vi "Demo_Single-Channel device.vi"() -> ()   [LabVIEW 2011]
doc: "This example shows how to configure a range and check that the acquired measurements are within that range using the VIs of the driver."
uses:
  <instrlib>/Thorlabs_MDT69xB/Thorlabs_MDT69xB.lvlib
panel:
  in  "Set x max Voltage(V)":dbl
  out "Get x min voltage(V)":dbl
  in  "Set x min Voltage(V)":dbl
  out "Get x max voltage(V)":dbl
  out "v limit(V)":dbl
  out "Get X voltage(V)":dbl
  in  "Set X voltage(V)":dbl
  out "?":string
  # "Device Info"
  # "Set Params"
  # "Get Params"
  # "(c) 2019 <Thorlabs>.  ALL RIGHTS RESERVED."
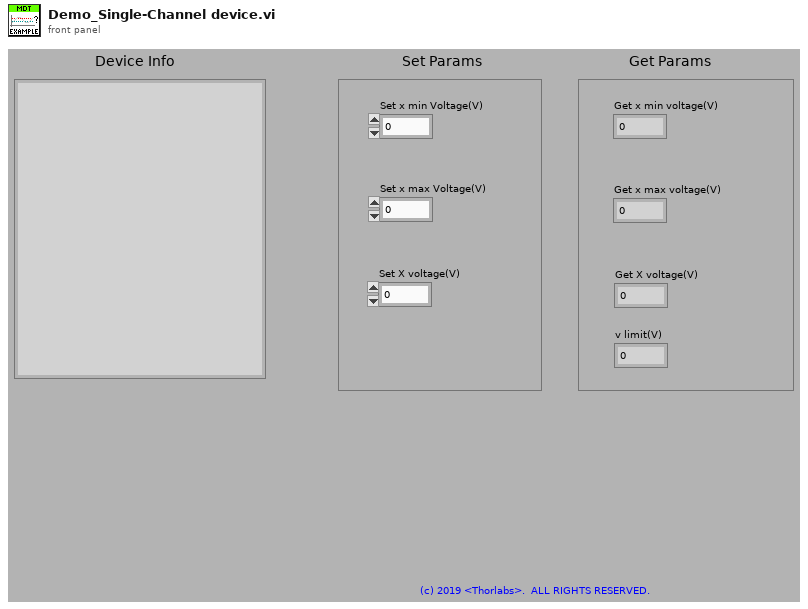
[diagram p1: front panel]
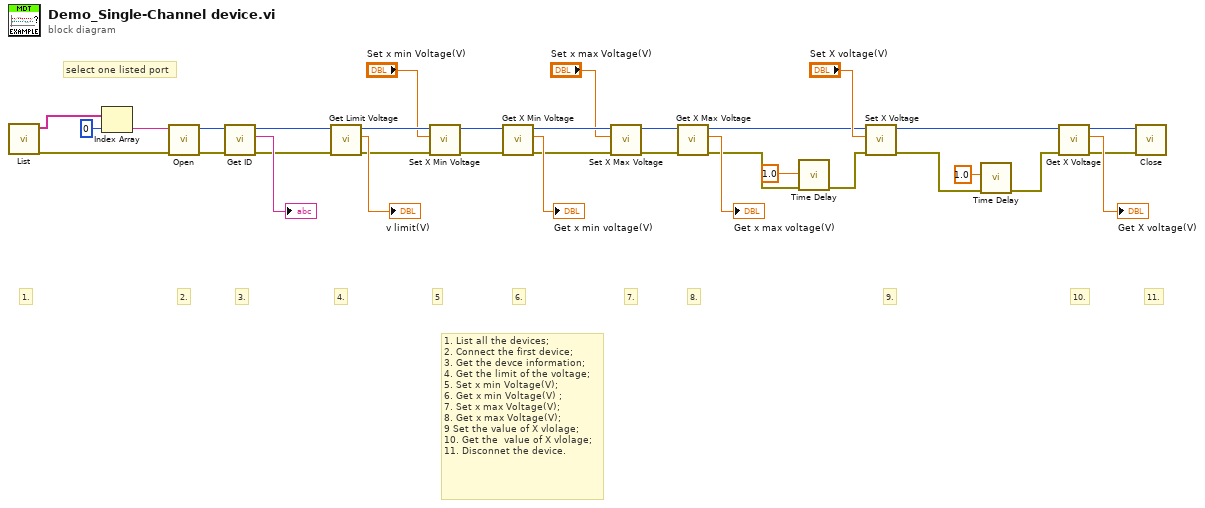
[diagram p0: block diagram]
diagram:
  # "10."
  # "9."
  # "8."
  # "7."
  # "6."
  # "5"
  # "1. List all the devices;\n2. Connect the first device;\n3. Get the devce information;\n4. Get the limit of the voltage;\n5. Set x min Voltage(V);\n6. Get x min Voltage(V) ;\n7. Set x max Voltage(V); \n8. Get x max Voltage(V);\n9 Set the value of X vlolage;\n10. Get the  value of X vlolage;\n11. Disconnet the device."
  # "11."
  # "4."
  # "3."
  # "2."
  # "1."
  # "select one listed port"
  n1 = call <instrlib>:"List.vi"() -> ("error out"=w30:errorcluster, "COM ports"=w33:string[])  [unwired: 10 in]
  n2 = Index Array(array=w33, index=0) -> (element=w31:string)
  n3 = call <instrlib>:"Open.vi"("error in (no error)"=w30, "Serial Port"=w31) -> ("error out"=w29:errorcluster, "hDevice"=w28:i32)  [unwired: 7 in, 1 out]
  n4 = call <instrlib>:"Get ID.vi"("error in (no error)"=w29, "hdl in"=w28) -> ("error out"=w16:errorcluster, "ID"=→"?":string, "hdl out"=w27:i32)  [unwired: 7 in]
  n5 = call <instrlib>:"Get Limit Voltage.vi"("error in (no error)"=w16, "hdl in"=w27) -> ("error out"=w7:errorcluster, "v limit"=→"v limit(V)":dbl, "hdl out"=w17:i32)  [unwired: 7 in]
  n6 = call <instrlib>:"Set X Min Voltage.vi"("error in (no error)"=w7, "Set x min Voltage(V)"="Set x min Voltage(V)", "hdl in"=w17) -> ("error out"=w6:errorcluster, "hdl"=w14:i32)  [unwired: 7 in]
  n7 = call <instrlib>:"Get X Min Voltage.vi"("error in (no error)"=w6, "hdl in"=w14) -> ("error out"=w5:errorcluster, "Get x min voltage(V)"=→"Get x min voltage(V)":dbl, "hdl"=w13:i32)  [unwired: 7 in]
  n8 = call <instrlib>:"Set X Max Voltage.vi"("error in (no error)"=w5, "Set x max Voltage(V)"="Set x max Voltage(V)", "hdl in"=w13) -> ("error out"=w4:errorcluster, "hdl"=w12:i32)  [unwired: 7 in]
  n9 = call <instrlib>:"Get X Max Voltage.vi"("error in (no error)"=w4, "hdl in"=w12) -> ("error out"=w2:errorcluster, "Get x max voltage(V)"=→"Get x max voltage(V)":dbl, "hdl"=w3:i32)  [unwired: 7 in]
  n10 = call "Time Delay"("error in (no error)"=w2, "Delay Time (s)"=1.0) -> ("error out"=w1:errorcluster)  [unwired: 9 in]
  n11 = call <instrlib>:"Set X Voltage.vi"("error in (no error)"=w1, "Set x Voltage(V)"="Set X voltage(V)", "hdl in"=w3) -> ("error out"=w26:errorcluster, "hdl"=w25:i32)  [unwired: 7 in]
  n12 = call "Time Delay"("error in (no error)"=w26, "Delay Time (s)"=1.0) -> ("error out"=w24:errorcluster)  [unwired: 9 in]
  n13 = call <instrlib>:"Get X Voltage.vi"("error in (no error)"=w24, "hdl in"=w25) -> ("error out"=w19:errorcluster, "Get x Voltage(V)"=→"Get X voltage(V)":dbl, "hdl"=w34:i32)  [unwired: 7 in]
  n14 = call <instrlib>:"Close.vi"("error in (no error)"=w19, "hDevice"=w34) -> ()  [unwired: 9 in, 1 out]
